vi "Construct String Control Sink.vi"(4 "Error Action":T1=enum."Ignore Error and Close Sink", 6 "Clear on Shutdown?(F)":bool, 7 "Str Refnum":refnum<vi>, 8 "Log Filter":refnum<class "ILogFilter.lvclass">, 9 "AutoScroll?(F)":bool, 10 "LogFormat":refnum<class "IStringFormat.lvclass">, 11 "LogLevel":T2) -> (3 "String Control Sink out":refnum<class "String Control Sink.lvclass">)   [LabVIEW 2017, in "String Control Sink.lvclass"]
doc: "--\nCopyright © 2017 Composed SystemsI All rights reserved.\n\nAuthor: Jon McBee <jon.mcbee@composed.io>\n\nThis library is provided \"AS IS\" ,WITHOUT WARRANTIES OR\nCONDITIONS OF ANY KIND, either express or implied.\n\nComposed Systems -- composed.io\n\nStream 0.0.1.1\nJon McBee - Composed Systems\nCopyright (c) 2017, Composed Systems"
uses:
  <vilib>/gpm_packages/@cs/event-logger/Source/String Control Sink/String Control Sink.lvclass
  C:/Program Files/National Instruments/LabVIEW 2017/vi.lib/gpm_packages/@cs/event-logger/Source/Composed Log/Log Sink/Log Sink.lvclass
  C:/Program Files/National Instruments/LabVIEW 2017/vi.lib/gpm_packages/@cs/event-logger/Source/String Log Sink/String Log Sink.lvclass
  <vilib>/gpm_packages/@cs/event-logger/Source/Composed Log/Types/Log Level.ctl
  <vilib>/gpm_packages/@cs/event-logger/Source/IStringFormat/IStringFormat.lvclass
  <vilib>/gpm_packages/@cs/event-logger/Source/Composed Log/ILogFilter/ILogFilter.lvclass
  <vilib>/gpm_packages/@cs/event-logger/Source/Composed Log/Log Sink/Sink Error Actions ENUM.ctl
  <vilib>/gpm_packages/@cs/event-logger/Source/String Control Sink/String Control Sink.lvclass/String Control Sink.ctl
  <vilib>/gpm_packages/@cs/event-logger/Source/Composed Log/Log Sink/Log Sink.lvclass/Log Sink.ctl
  <vilib>/gpm_packages/@cs/event-logger/Source/String Log Sink/String Log Sink.lvclass/String Log Sink.ctl
  <vilib>/gpm_packages/@cs/event-logger/Source/Composed Log/Log Sink/Log Sink.lvclass
  <vilib>/gpm_packages/@cs/event-logger/Source/String Log Sink/String Log Sink.lvclass
  <vilib>/gpm_packages/@cs/event-logger/Source/Composed Log/Composed Log.lvlib
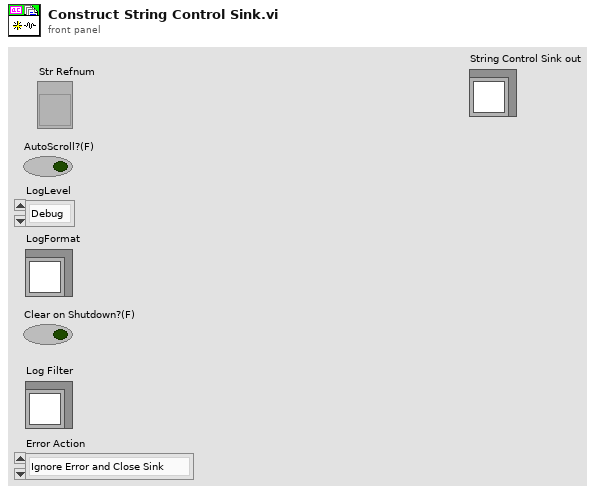
[diagram p1: front panel]
types:
  T1 = typedef "Composed Log.lvlib/Log Sink.lvclass/Sink Error Actions ENUM.ctl" = enum16{"Ignore Error and Continue", "Ignore Error and Close Sink", "Report Error and Close Sink"}
  T2 = typedef "Composed Log.lvlib/Log Level.ctl" = enum16{"Debug", "Info", "Warning", "Error", "Critical"}
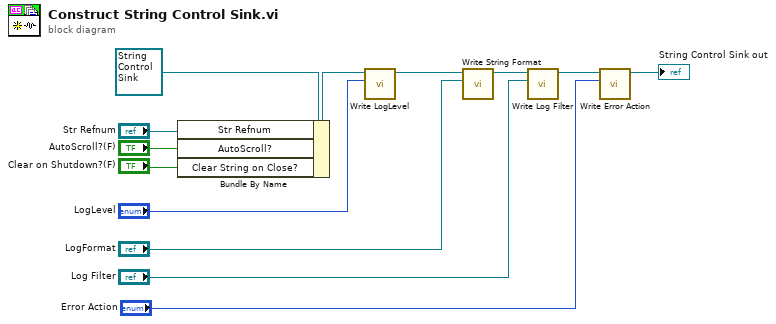
[diagram p0: block diagram]
diagram:
  n1 = Bundle By Name(cluster=refnum<class "String Control Sink.lvclass"> refnum ("String Control Sink in"), "Str Refnum"="Str Refnum", "AutoScroll?"="AutoScroll?(F)", "Clear String on Close?"="Clear on Shutdown?(F)") -> (w11:refnum<class "String Control Sink.lvclass">)
  n2 = call <vilib>:"Write LogLevel.vi"("LogLevel"="LogLevel", "Log Sink in"=w11) -> ("Log Sink out"=w9:refnum<class "String Control Sink.lvclass">)  [unwired: 8 in, 1 out]
  n3 = call <vilib>:"Write String Format.vi"("StringFormat"="LogFormat", "String Log Sink in"=w9) -> ("String Log Sink out"=w5:refnum<class "String Control Sink.lvclass">)  [unwired: 8 in, 1 out]
  n4 = call <vilib>:"Write Log Filter.vi"("Log Filter"="Log Filter", "Log Sink in"=w5) -> ("Log Sink out"=w3:refnum<class "String Control Sink.lvclass">)  [unwired: 8 in, 1 out]
  n5 = call <vilib>:"Write Error Action.vi"("Error Action"="Error Action", "Log Sink in"=w3) -> ("Log Sink out"=→"String Control Sink out":refnum<class "String Control Sink.lvclass">)  [unwired: 8 in, 1 out]
